vi "Actor Core.vi"(8 "error in":errorcluster, 11 "Nested in":refnum<class "Laser Oxxius Controller.lvclass">) -> (0 "error out":errorcluster, 3 "Actor out":refnum<class "Actor.lvclass">)   [LabVIEW 2020, in "Laser_Oxxius.lvlib" / "Laser Oxxius Controller.lvlib" / "Laser Oxxius Controller.lvclass"]
doc: "(<B>Filename</B>: Actor Framework.lvlib:Actor.lvclass:Actor Core.vi)\n\nReceives messages to the actor, reacts to them, and initiates any error handling that may shut the actor down.\n\nDescendant classes may override this VI to append parallel tasks for the actor to complete while it handles messages. Overrides use the Call Parent Method node."
uses:
  Laser Oxxius Controller.lvclass
  C:/Program Files/National Instruments/LabVIEW 2020/vi.lib/ActorFramework/Actor/Actor.lvclass
  <vilib>/ActorFramework/Actor/Actor.lvclass
  Laser Oxxius Controller.lvclass/Laser Oxxius Controller.ctl
  <vilib>/ActorFramework/Actor/Actor.lvclass/Actor.ctl
  <vilib>/ActorFramework/Message Enqueuer/Message Enqueuer.lvclass/Message Enqueuer.ctl
  Laser_Oxxius/Laser_Oxxius Messages/SetPower Msg/SetPower Msg.lvclass/SetPower Msg.ctl
  Laser_Oxxius/Laser_Oxxius Messages/SetShutterStatus Msg/SetShutterStatus Msg.lvclass/SetShutterStatus Msg.ctl
  Laser_Oxxius/Laser_Oxxius Messages/SetAutoShutter Msg/SetAutoShutter Msg.lvclass/SetAutoShutter Msg.ctl
  <vilib>/ActorFramework/Message Enqueuer/Init from Existing Queue.vi
  <vilib>/ActorFramework/Message Enqueuer/Enqueue.vi
  Laser_Oxxius/Laser_Oxxius Messages/SetPower Msg/SetPower Msg.lvclass
  C:/Program Files/National Instruments/LabVIEW 2020/vi.lib/ActorFramework/Message/Message.lvclass
  Laser_Oxxius/Laser_Oxxius Messages/SetShutterStatus Msg/SetShutterStatus Msg.lvclass
  Laser_Oxxius/Laser_Oxxius Messages/SetAutoShutter Msg/SetAutoShutter Msg.lvclass
  <vilib>/ActorFramework/Stop Msg/Stop Msg.lvclass
  <vilib>/ActorFramework/Message Priority Queue/Priority Enqueue.vi
  <vilib>/ActorFramework/Message Enqueuer/Message Enqueuer.lvclass
panel:
  in  "405 Auto":bool caption="LAS-05997"
  in  "488 Auto":bool caption="LAS-06030"
  in  "532 Auto":bool caption="LAS-05886"
  in  "561 Auto":bool caption="LAS-05858"
  in  "647 Auto":bool caption="LAS-05914"
  in  "785 Auto":bool caption="LAS-03914"
  in  "785 Power":dbl caption="LAS-03914" min=0.0 max=200.0
  in  "785":bool caption="LAS-03914"
  in  "647 Power":sgl caption="LAS-05914"
  in  "647":bool caption="LAS-05914"
  in  "561 Power":dbl caption="LAS-05858" min=0.0 max=200.0
  in  "561":bool caption="LAS-05858"
  in  "532 Power":sgl caption="LAS-05886" min=0 max=200
  in  "532":bool caption="LAS-05886"
  in  "488 Power":dbl caption="LAS-06030" min=0.0 max=200.0
  in  "488":bool caption="LAS-06030"
  in  "405 Power":dbl caption="LAS-05997" min=0.0 max=200.0
  in  "405":bool caption="LAS-05997"
  # "Power(%)"
  # "On/Off"
  # "AutoShutter"
  # "Lasers"
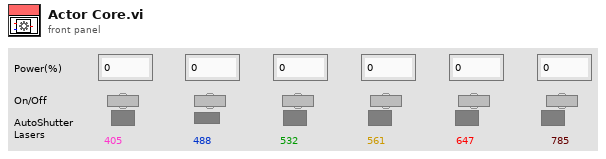
[diagram p1: front panel]
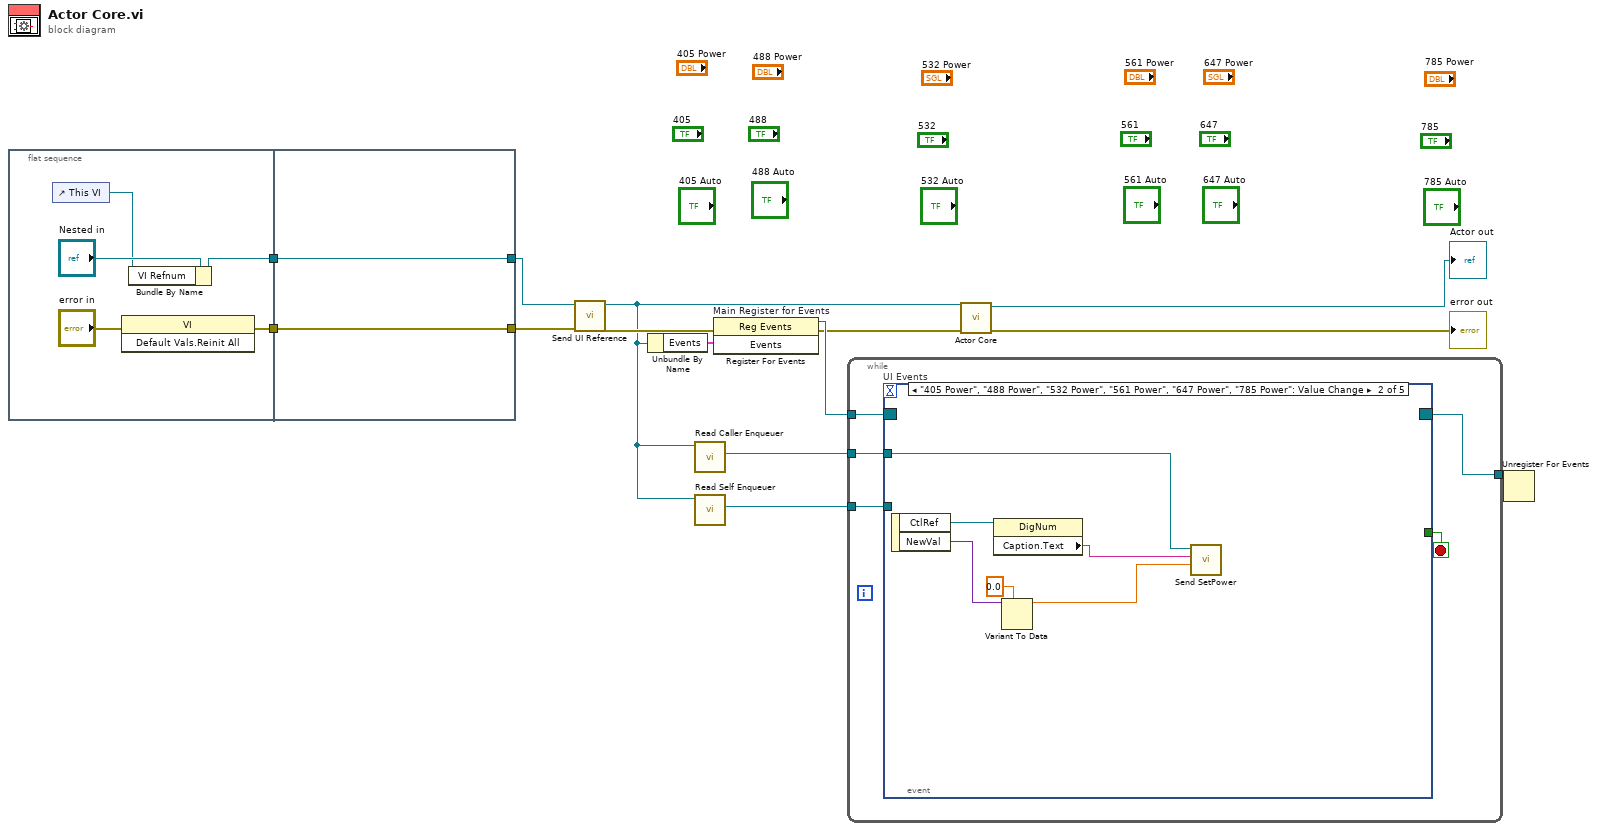
[diagram p0: block diagram]
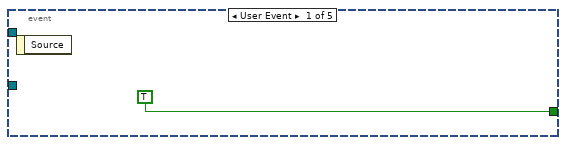
[diagram p2: hidden frame]
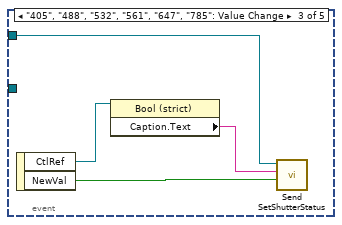
[diagram p3: hidden frame]
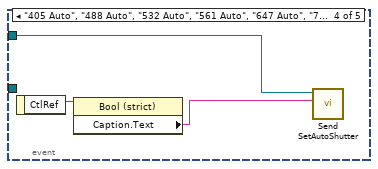
[diagram p4: hidden frame]
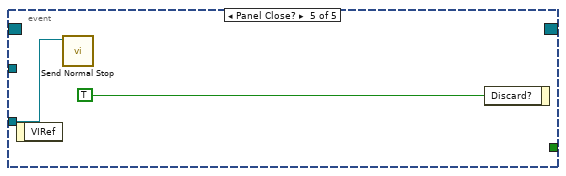
[diagram p5: hidden frame]
diagram:
  n1 = flat-sequence {
    tunnel: [w17] -> w6
    tunnel: [w16] -> w5
    tunnel: [w20] -> w2
    tunnel: [w21] -> w7
    tunnel: w6 -> [w21]
    tunnel: w5 -> [w20]
    frame #0 {
      n2 = control-ref of="This VI"() -> (w15:refnum<vi>)
      n3 = invoke class="VI" method="Default Vals.Reinit All"(error in="error in") -> (error out=w17:errorcluster)  [unwired: 2 in, 2 out]
      n4 = Bundle By Name(cluster="Nested in", "VI Refnum"=w15) -> (w16:refnum<class "Laser Oxxius Controller.lvclass">)
    }
    frame #1 {
    }
  }
  n5 = call-dynamic "Send UI Reference.vi"("error in (no error)"=w7, "Laser Oxxius Controller in"=w2) -> ("error out"=w3:errorcluster, "Laser Oxxius Controller out"=w1:refnum<class "Laser Oxxius Controller.lvclass">)  [unwired: 8 in]
  n6 = Unbundle By Name(w1) -> ("Events"=w11:cluster{"Stop":refnum<user-event>})
  n7 = call <vilib>:"Read Caller Enqueuer.vi"("Actor"=w1) -> ("Caller Enqueuer"=w4:refnum<class "Message Enqueuer.lvclass">)  [unwired: 10 in]
  n8 = call <vilib>:"Read Self Enqueuer.vi"("Actor"=w1) -> ("Self Enqueuer"=w9:refnum<class "Message Enqueuer.lvclass">)  [unwired: 10 in]
  n9 = register-events "Main Register for Events"(error in=w3, w11) -> (reference out=w12:refnum<event-registration>, error out=w8:errorcluster)  [unwired: 1 in]
  n10 = while {
    tunnel: w12 -> [w26]
    tunnel: [w24] -> w10
    tunnel: w9 -> [w23]
    tunnel: w4 -> [w22]
    stop <- w25 stop-if-true
    n11 = event "UI Events" shown="[1] \"405 Power\", \"488 Power\", \"532 Power\", \"561 Power\", \"647 Power\", \"785 Power\": Value Change" {
      selector: w26 -> [_ _ _ _ _]
      dyn-events: [_ _ _ _ _] -> w24
      timeout: _ -> [_ _ _ _ _]
      tunnel: [TRUE _ _ _ _] -> w25
      tunnel: w23 -> [_ _ _ _ w41]
      tunnel: w22 -> [_ w33 w37 w40 _]
      event User Event {
        n12 = event-data() -> ()  [unwired: 1 in, 1 out]
      }
      event "405 Power", "488 Power", "532 Power", "561 Power", "647 Power", "785 Power": Value Change {
        n13 = event-data() -> ("CtlRef"=w32:refnum<vi>, "NewVal"=w30:variant)  [unwired: 1 in]
        n14 = property class="DigNum"(reference=w32) -> ("Caption.Text"=w31:string)  [unwired: 1 in, 2 out]
        n15 = Variant To Data(type=0.0 ("Value"), Variant=w30) -> (data=w28:dbl)  [unwired: 1 in, 1 out]
        n16 = call "Send SetPower.vi"("Value"=w28, "Label"=w31, "Message Enqueuer"=w33) -> ()  [unwired: 7 in, 2 out]
      }
      event "405", "488", "532", "561", "647", "785": Value Change {
        n17 = event-data() -> ("CtlRef"=w36:refnum<vi>, "NewVal"=w34:bool)  [unwired: 1 in]
        n18 = property class="Bool (strict)"(reference=w36) -> ("Caption.Text"=w35:string)  [unwired: 1 in, 2 out]
        n19 = call "Send SetShutterStatus.vi"("Value"=w34, "Label"=w35, "Message Enqueuer"=w37) -> ()  [unwired: 7 in, 2 out]
      }
      event "405 Auto", "488 Auto", "532 Auto", "561 Auto", "647 Auto", "785 Auto": Value Change {
        n20 = event-data() -> ("CtlRef"=w39:refnum<vi>)  [unwired: 1 in]
        n21 = property class="Bool (strict)"(reference=w39) -> ("Caption.Text"=w38:string)  [unwired: 1 in, 2 out]
        n22 = call "Send SetAutoShutter.vi"("Label"=w38, "Message Enqueuer"=w40) -> ()  [unwired: 8 in, 2 out]
      }
      event Panel Close? {
        n23 = event-data() -> ()  [unwired: 1 in, 1 out]
        n24 = call <vilib>:"Send Normal Stop.vi"("Message Enqueuer"=w41) -> ()  [unwired: 10 in, 1 out]
        n25 = event-data("Discard?"=TRUE) -> ()  [unwired: 1 in, 1 out]
      }
    }
  }
  n26 = call-parent "Actor Core.vi"("error in"=w8, "Actor in"=w1) -> ("error out"=→"error out":errorcluster, "Actor out"=→"Actor out":refnum<class "Actor.lvclass">)  [unwired: 8 in]
  n27 = Unregister For Events(event registration refnum=w10) -> ()  [unwired: 1 in, 1 out]
